vi "unsubscribe.vi"(8 "error in":errorcluster, 10 "command":string, 11 "refnum in":T1) -> (0 "error out":errorcluster, 3 "refnum in":T1)   [LabVIEW 2020, in "Publisher Subscriber.lvlib"]
uses:
  Publisher Subscriber.lvlib
  Controls/node refnum.ctl
  Controls/node dvr data.ctl
  Controls/data cluster.ctl
  Controls/subscription bank ref.ctl
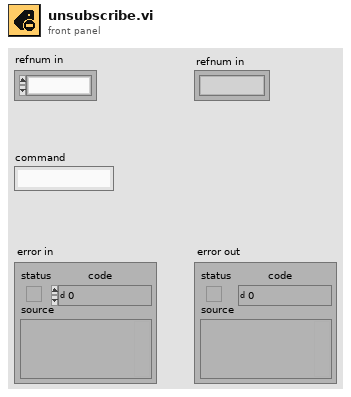
[diagram p1: front panel]
types:
  T1 = typedef "Publisher Subscriber.lvlib/node refnum.ctl" = refnum<k1>
  T2 = typedef "Publisher Subscriber.lvlib/node dvr data.ctl" = cluster{"queue ref":refnum<queue>, "Subscription Bank Ref":refnum<data-value>, "Command":string, "Data":variant, "Subscriptions []":set{string}, "Variables DVR Ref":refnum<data-value>}
  T3 = typedef "Publisher Subscriber.lvlib/subscription bank ref.ctl" = map{string, set{refnum<queue>}}
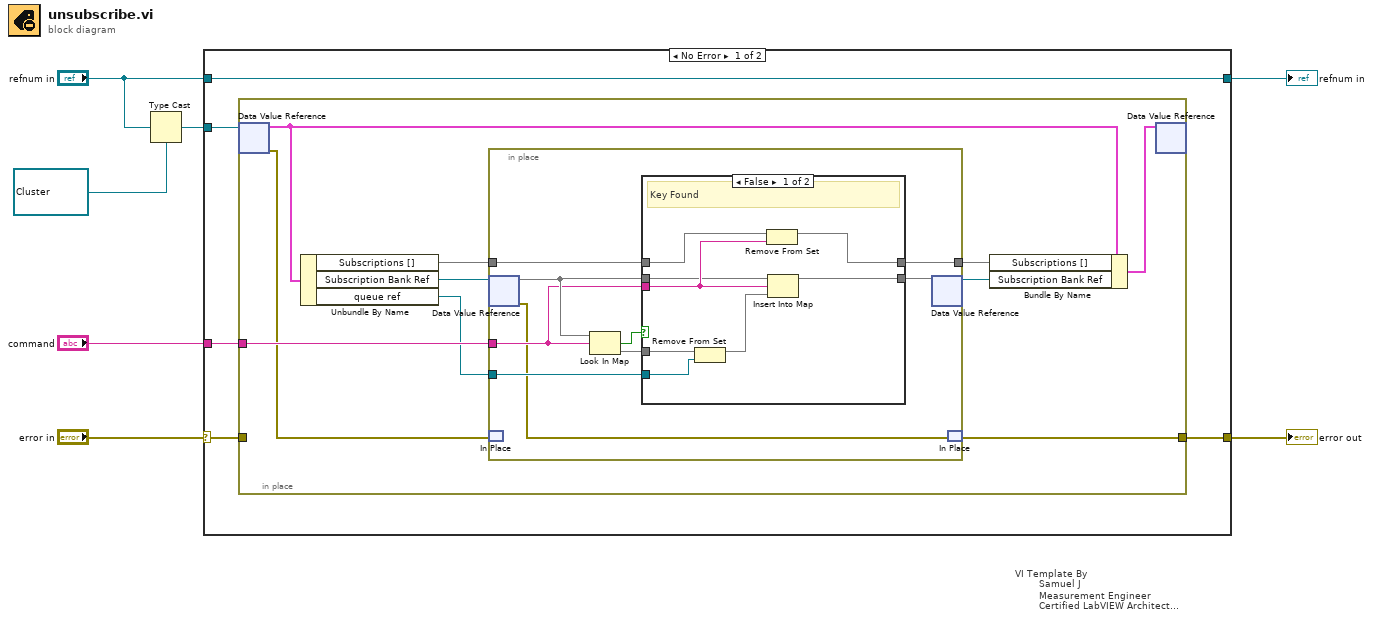
[diagram p0: block diagram]
diagram:
  n1 = Type Cast(type=refnum<data-value> refnum ("data value reference"), x="refnum in") -> (*(type *) &x=w3:refnum<data-value>)
  n2 = case "VI Template By\n        Samuel J\n        Measurement Engineer\n        Certified LabVIEW Architect\n        Vestas Technology R&D Chennai" shown="No Error" "error in" {
    selector: "error in" -> [w9 w43]
    tunnel: [w8 w43] -> w6
    tunnel: "command" -> [w10 _]
    tunnel: w3 -> [w11 _]
    tunnel: [w12 w42] -> w2
    tunnel: "refnum in" -> [w12 w42]
    frame No Error {
      n3 = in-place {
        in-place-border: w10 -> [w19]
        in-place-border: [w14] -> w8
        in-place-border: w9 -> [_]
        n4 = in-place-dvr #1(w11) -> (w21:T2, w13:errorcluster)
        n5 = Unbundle By Name(w21) -> ("Subscriptions []"=w16:set{string}, "Subscription Bank Ref"=w20:refnum<data-value>, "queue ref"=w17:refnum<queue>)
        n6 = in-place {
          in-place-border: w19 -> [w28]
          in-place-border: w17 -> [w29]
          in-place-border: w16 -> [w27]
          in-place-border: [w26] -> w15
          n7 = in-place-dvr #2(w20) -> (w31:T3, w25:errorcluster)
          n8 = in-place-match #3(w13) -> ()  [unwired: 1 out]
          n9 = Look In Map(map=w31, key=w28) -> (key not found?=w24:bool, value=w23:set{refnum<queue>})  [unwired: 1 in]
          n10 = case shown="False" w24 {
            tunnel: w23 -> [w39 _]
            tunnel: w31 -> [w33 w40]
            tunnel: [w32 w40] -> w30
            tunnel: w29 -> [w38 _]
            tunnel: w28 -> [w35 _]
            tunnel: w27 -> [w37 w41]
            tunnel: [w34 w41] -> w26
            frame False {
              # "Key Found"
              n11 = Remove From Set(10:w38, 11:w39) -> (3:w36:set{refnum<queue>})  [unwired: 1 out]
              n12 = Remove From Set(10:w35, 11:w37) -> (3:w34:set{string})  [unwired: 1 out]
              n13 = Insert Into Map(map in=w33, key=w35, value=w36) -> (map out=w32:T3)  [unwired: 2 out]
            }
            frame True {
              # "Key Not Found"
            }
          }
          n14 = in-place-dvr #2(w30) -> (w18:refnum<data-value>)  [unwired: 1 out]
          n15 = in-place-match #3(w25) -> (w14:errorcluster)
        }
        n16 = Bundle By Name(cluster=w21, "Subscriptions []"=w15, "Subscription Bank Ref"=w18) -> (w22:T2)
        n17 = in-place-dvr #1(w22) -> ()  [unwired: 2 out]
      }
    }
    frame Error {
    }
  }
  "error out" <- w6
  "refnum in" <- w2
